vi "ColumnSort.vi"(8 "error in (no error)":errorcluster, 9 "Desend":bool, 11 "MCListbox Refnum":refnum<vi>) -> (0 "error out":errorcluster)   [LabVIEW 2011]
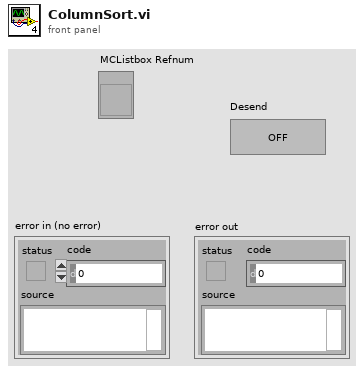
[diagram p1: front panel]
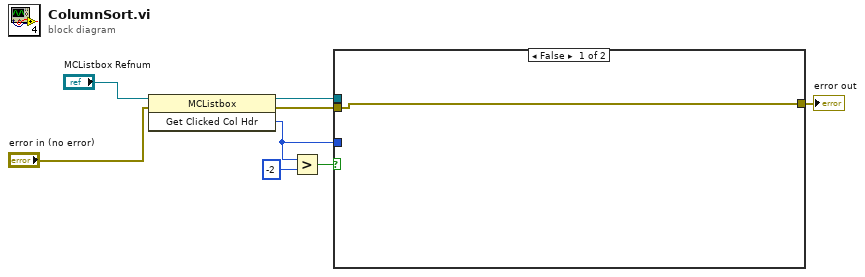
[diagram p0: block diagram]
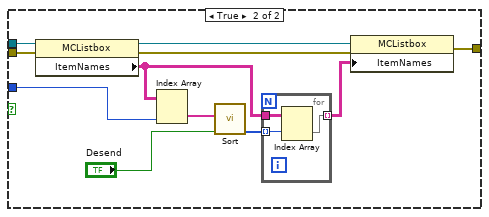
[diagram p2: hidden frame]
diagram:
  n1 = invoke class="MCListbox" method="Get Clicked Col Hdr"(reference="MCListbox Refnum", error in="error in (no error)") -> (reference out=w5:refnum<vi>, error out=w4:errorcluster, "Get Clicked Column Header"=w3:i32)  [unwired: 1 in]
  n2 = Greater?(x=w3, y=-2) -> (0:w7:bool)
  n3 = case shown="False" w7 {
    tunnel: w5 -> [_ w19]
    tunnel: w4 -> [w9 w20]
    tunnel: w3 -> [_ w18]
    tunnel: [w9 w10] -> w2
    frame False {
    }
    frame True {
      n4 = property class="MCListbox"(reference=w19, error in=w20) -> (reference out=w15:refnum<vi>, error out=w14:errorcluster, "ItemNames"=w12:string[][])
      n5 = Index Array(array=w12, index (col)=w18) -> (element=w17:string[])  [unwired: 1 in]
      n6 = call "Sort.vi"("desend"="Desend", "Array"=w17) -> ("sorted Index"=w13:i32[])  [unwired: 8 in, 1 out]
      n7 = for {
        tunnel: w13 -> [w23] mode=indexing
        tunnel: [w22] -> w11 mode=indexing
        tunnel: w12 -> [w21]
        n8 = Index Array(array=w21, index (row)=w23) -> (element=w22:string[])  [unwired: 1 in]
      }
      n9 = property class="MCListbox"(reference=w15, error in=w14, "ItemNames"=w11) -> (error out=w10:errorcluster)  [unwired: 1 out]
    }
  }
  "error out" <- w2
